vi "Configure List Step Count.vi"(8 "error in (no error)":errorcluster, 10 "List Total":i32=1 min=0, 11 "VISA resource name":refnum<visa-resource-name>) -> (0 "error out":errorcluster, 3 "VISA resource name out":refnum<visa-resource-name>)   [LabVIEW 2015, in "IT6700H.lvlib"]
doc: "Configure the number of steps in a list."
uses:
  <instrlib>/IT6700H/IT6700H.lvlib
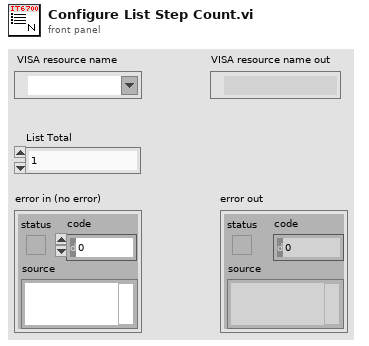
[diagram p1: front panel]
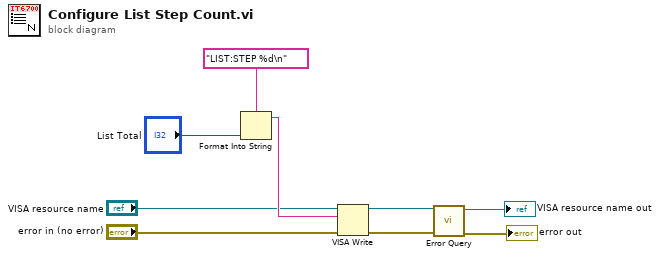
[diagram p0: block diagram]
diagram:
  n1 = Format Into String(format string="LIST:STEP %d\n", "List Total") -> (resulting string=w7:string)  [unwired: 2 in, 1 out]
  n2 = VISA Write(VISA resource name="VISA resource name", write buffer=w7, error in (no error)="error in (no error)") -> (VISA resource name out=w3:refnum<visa-resource-name>, error out=w4:errorcluster)  [unwired: 1 out]
  n3 = call <instrlib>:"Error Query.vi"("error in (no error)"=w4, "VISA resource name"=w3) -> ("error out"=→"error out":errorcluster, "VISA resource name out"=→"VISA resource name out":refnum<visa-resource-name>)  [unwired: 6 in, 2 out]
